vi "parse.total.pagination.vi"(7 "series body":string, 8 "error in (no error)":errorcluster, 11 "ComicVine_class in":refnum<class "series_class.lvclass">) -> (0 "error out":errorcluster, 2 "paginated count":i32, 3 "ComicVine_class out":refnum<class "series_class.lvclass">)   [LabVIEW 2024, in "series_class.lvclass"]
uses:
  series_class.lvclass
  series_class.lvclass/series_class.ctl
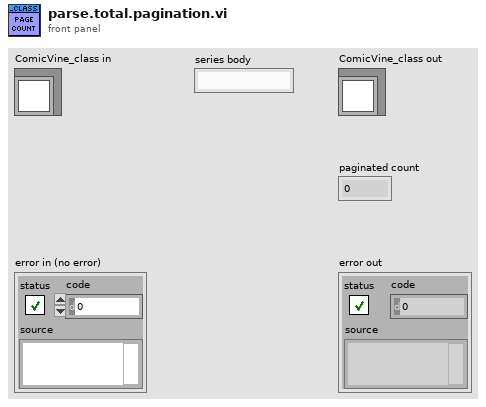
[diagram p1: front panel]
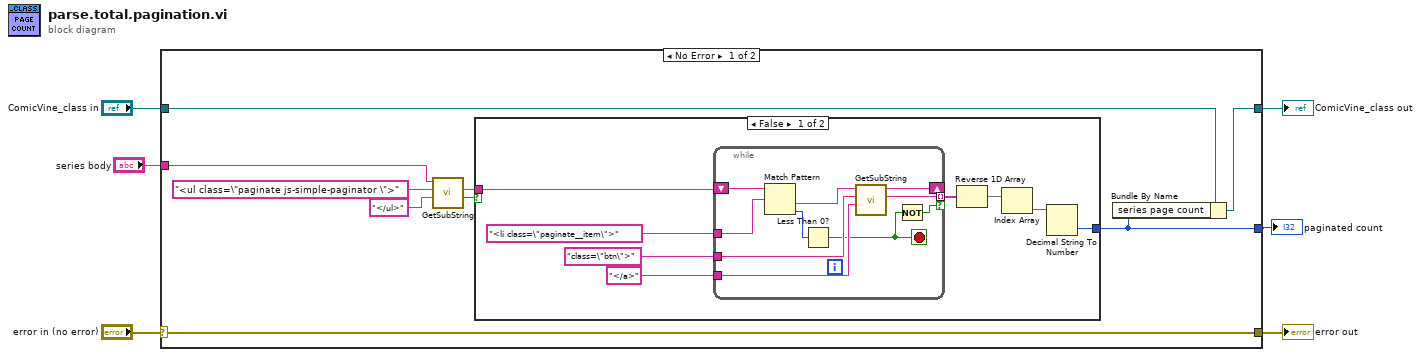
[diagram p0: block diagram]
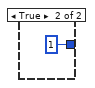
[diagram p2: hidden frame]
diagram:
  n1 = case shown="No Error" "error in (no error)" {
    selector: "error in (no error)" -> [w15 w36]
    tunnel: [w15 w36] -> w5
    tunnel: [w12 w35] -> w3
    tunnel: "ComicVine_class in" -> [w14 w35]
    tunnel: [w13 _] -> w2
    tunnel: "series body" -> [w7 _]
    frame No Error {
      n2 = call "GetSubString.vi"("End Search"="</ul>", "Start Search"="<ul class=\"paginate js-simple-paginator \">", "String In"=w7) -> ("Not Found?"=w9:bool, "Match"=w8:string)  [unwired: 6 in, 1 out]
      n3 = case shown="False" w9 {
        tunnel: [w18 1] -> w13
        tunnel: w8 -> [w16 _]
        frame False {
          n4 = while {
            shift-right: [w33] -> _
            shift-left: w16 -> [w28]
            tunnel: "class=\"btn\">" -> [w32]
            tunnel: "</a>" -> [w31]
            tunnel: [w30] -> w21 mode=indexing if=w29
            tunnel: "<li class=\"paginate__item\">" -> [w26]
            stop <- w24 stop-if-true
            n5 = Match Pattern(string=w28, regular expression=w26) -> (after substring=w27:string, offset past match=w25:i32)  [unwired: 1 in, 2 out]
            n6 = Less Than 0?(x=w25) -> (x < 0?=w24:bool)
            n7 = call "GetSubString.vi"("End Search"=w31, "Start Search"=w32, "String In"=w27) -> ("Match"=w30:string, "Following String Out"=w33:string)  [unwired: 6 in, 1 out]
            n8 = Not(x=w24) -> (.not. x?=w29:bool)
          }
          n9 = Reverse 1D Array(array=w21) -> (reversed array=w20:string[])
          n10 = Index Array(array=w20) -> (element=w19:string)  [unwired: 1 in]
          n11 = Decimal String To Number(string=w19) -> (number=w18:i32)  [unwired: 2 in, 1 out]
        }
        frame True {
        }
      }
      n12 = Bundle By Name(cluster=w14, "series page count"=w13) -> (w12:refnum<class "series_class.lvclass">)
    }
    frame Error {
    }
  }
  "error out" <- w5
  "ComicVine_class out" <- w3
  "paginated count" <- w2
